vi "Initialization.vi"() -> (2 "Deviceindex":i32, 3 "Initialization Status":string, 4 "DLL Version":string, 5 "Initialization Error":bool)   [LabVIEW 2019]
uses:
  phlib.dll
panel:
  in  "String5[8]":string="**********"
  out "Serial[8]":string="**********"
  in  "String2[8]":string="**********"
  in  "String4[8]":string="**********"
  in  "String1[8]":string="**********"
  out "Returncode PH_Initialize":i32
  in  "String3[16]":string="*****************"
  out "Returncode PH_GetHardwareVersion":i32
  # "Warning: Do not change\nString initialization for required size!"
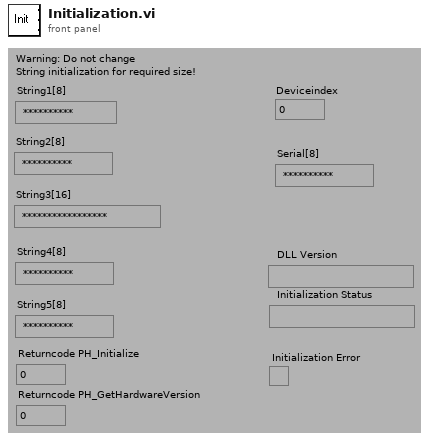
[diagram p1: front panel]
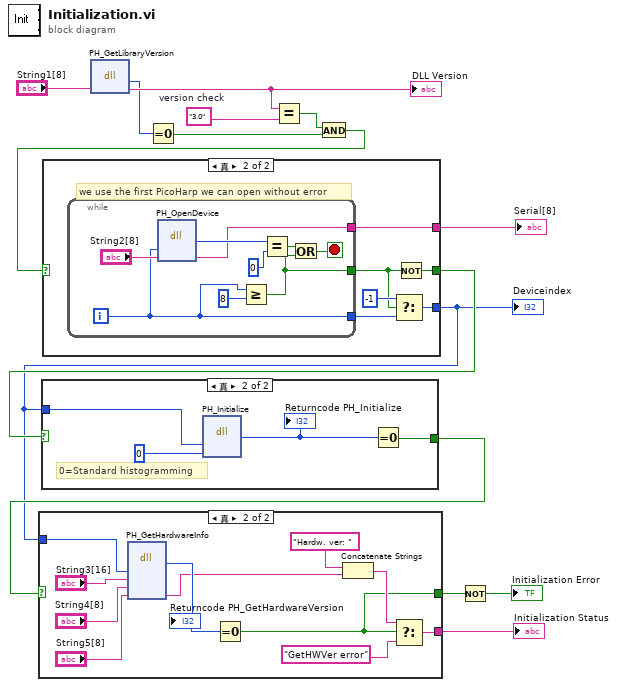
[diagram p0: block diagram]
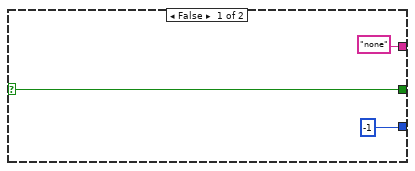
[diagram p2: hidden frame]
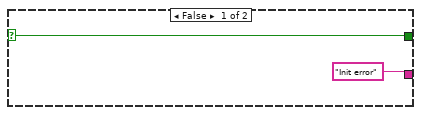
[diagram p4: hidden frame]
diagram:
  w9 = "3.0"  # version check
  n1 = dll-call lib="phlib.dll" fn="PH_GetLibraryVersion"("Version"="String1[8]") -> (w5:i32, "Version"=w10:string)  [unwired: 3 in, 2 out]
  "DLL Version" <- w10
  n2 = Equal To 0?(x=w5) -> (x = 0?=w6:bool)
  n3 = Equal?(x=w10, y=w9) -> (x = y?=w7:bool)
  n4 = And(x=w7, y=w6) -> (x .and. y?=w4:bool)
  n5 = case shown="真" w4 {
    selector: w4 -> [w17 _]
    tunnel: [w17 w19] -> w3
    tunnel: [-1 w22] -> w2
    tunnel: ["none" w18] -> w1
    frame False {
    }
    frame True {
      # "we use the first PicoHarp we can open without error"
      n6 = while {
        tunnel: [w24] -> w18
        tunnel: [w28] -> w23
        tunnel: [w26] -> w20
        i -> [w28]
        stop <- w25 stop-if-true
        n7 = dll-call lib="phlib.dll" fn="PH_OpenDevice"("devidx"=w28, "serial"="String2[8]") -> (w30:i32, "serial"=w24:string)  [unwired: 4 in, 2 out]
        n8 = Greater Or Equal?(x=w28, y=8) -> (x >= y?=w26:bool)
        n9 = Equal?(x=w30, y=0) -> (x = y?=w27:bool)
        n10 = Or(x=w27, y=w26) -> (x .or. y?=w25:bool)
      }
      n11 = Select(t=-1, s=w20, f=w23) -> (s? t:f=w22:i32)
      n12 = Not(x=w20) -> (.not. x?=w19:bool)
    }
  }
  "Deviceindex" <- w2
  "Serial[8]" <- w1
  n13 = case shown="真" w3 {
    selector: w3 -> [w33 _]
    tunnel: [w33 w36] -> w8
    tunnel: w2 -> [_ w35]
    frame False {
    }
    frame True {
      # "0=Standard histogramming"
      n14 = dll-call lib="phlib.dll" fn="PH_Initialize"("devidx"=w35, "mode"=0) -> (w37:i32)  [unwired: 5 in, 2 out]
      "Returncode PH_Initialize" <- w37
      n15 = Equal To 0?(x=w37) -> (x = 0?=w36:bool)
    }
  }
  n16 = case shown="真" w8 {
    selector: w8 -> [w38 _]
    tunnel: ["Init error" w46] -> w14
    tunnel: [w38 w45] -> w12
    tunnel: w2 -> [_ w44]
    frame False {
    }
    frame True {
      n17 = dll-call lib="phlib.dll" fn="PH_GetHardwareInfo" label="PH_GetHardwareVersion"("devidx"=w44, "Model"="String3[16]", "Partnum"="String4[8]", "Version"="String5[8]") -> (w48:i32, "Version"=w40:string)  [unwired: 6 in, 2 out]
      "Returncode PH_GetHardwareVersion" <- w48
      n18 = Equal To 0?(x=w48) -> (x = 0?=w45:bool)
      n19 = Concatenate Strings("Hardw. ver: ", w40) -> (w50:string)
      n20 = Select(t=w50, s=w45, f="GetHWVer error") -> (s? t:f=w46:string)
    }
  }
  "Initialization Status" <- w14
  n21 = Not(x=w12) -> (.not. x?=→"Initialization Error":bool)
